vi "T_step_Kelvinox.vi"   [LabVIEW 2019]
uses:
  Global/Global Variables/global.vi
  Instrument_Setup.vi
  Global/Global Variables/Data_Display_global.vi
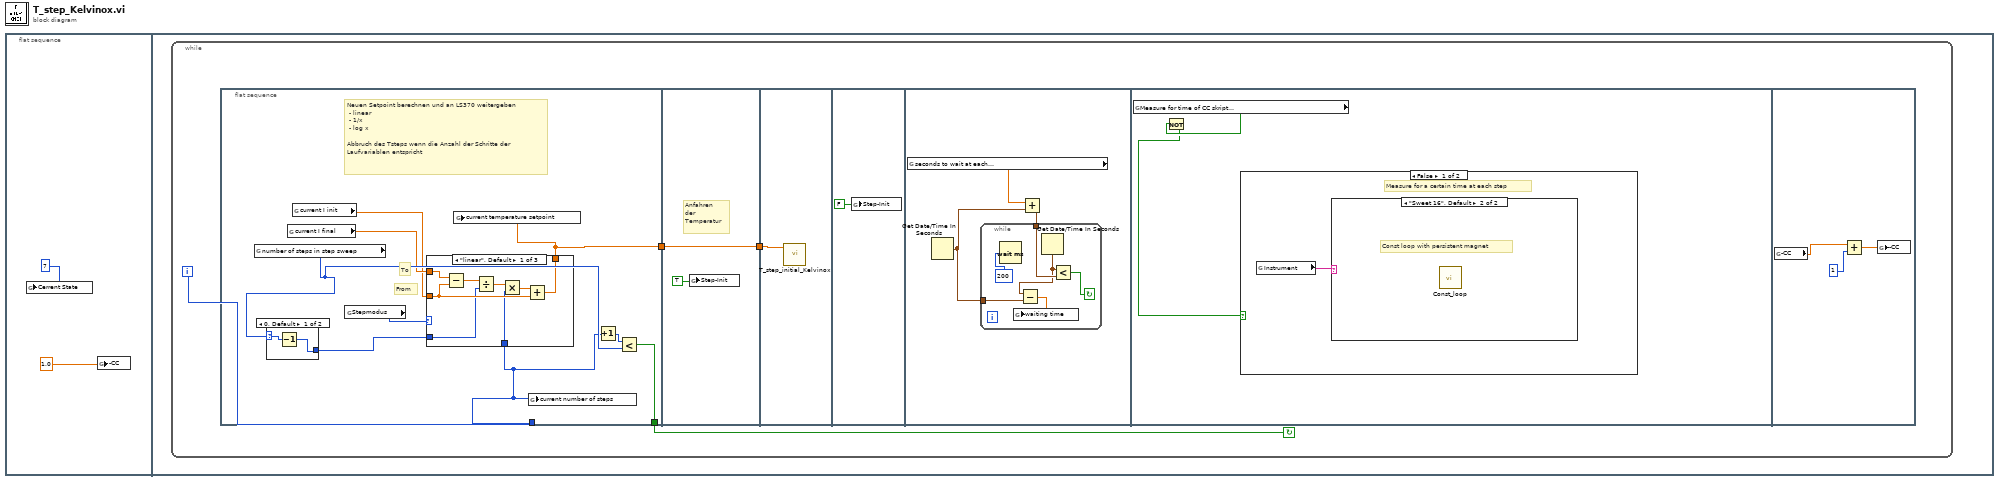
[diagram p0: block diagram]
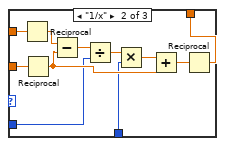
[diagram p3: hidden frame]
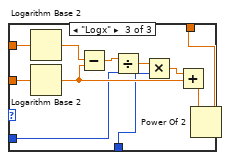
[diagram p4: hidden frame]
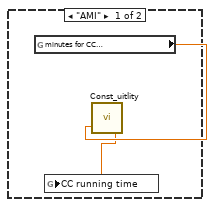
[diagram p5: hidden frame]
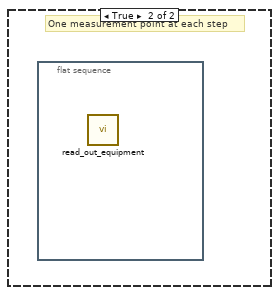
[diagram p6: hidden frame]
diagram:
  n1 = flat-sequence {
    frame #0 {
      n2 = global write "global.vi" "Cerrent State"(7) -> ()
      n3 = global write "global.vi" "-CC"(1.0) -> ()
    }
    frame #1 {
      n4 = while {
        i -> [w6]
        stop <- w5 continue-if-true
        n5 = flat-sequence {
          tunnel: w6 -> [w8]
          tunnel: [w9] -> w5
          tunnel: [w7] -> w3
          tunnel: [w49] -> w4
          tunnel: w3 -> [w49]
          tunnel: w4 -> [w51]
          frame #0 {
            # "Neuen Setpoint berechnen und an LS370 weitergeben\n - linear\n - 1/x\n - log x\n\nAbbruch des Tsteps wenn die Anzahl der Schritte der \nLaufvariablen entspricht"
            # "From"
            # "To"
            n6 = global read "global.vi" "number of steps in step sweep"() -> (w13:i32)
            n7 = case shown="0, Default" w13 {
              selector: w13 -> [w17 w18]
              tunnel: [w16 w18] -> w14
              frame 0, Default {
                n8 = Decrement(x=w17) -> (x-1=w16:i32)
              }
              frame 1 {
              }
            }
            n9 = global read "global.vi" "current I final"() -> (w11:dbl)
            n10 = global read "global.vi" "current I init"() -> (w10:dbl)
            n11 = global read "Instrument_Setup.vi" "Stepmodus"() -> (w12:enum16{"linear", "1/x", "Logx"})
            n12 = case shown="\"linear\", Default" w12 {
              tunnel: w11 -> [w26 w36 w48]
              tunnel: w10 -> [w23 w37 w47]
              tunnel: [w21 w31 w40] -> w7
              tunnel: w14 -> [w20 w28 w39]
              tunnel: w8 -> [w19 w27 w38]
              frame "linear", Default {
                n13 = Subtract(x=w26, y=w23) -> (x-y=w25:dbl)
                n14 = Divide(x=w25, y=w20) -> (x/y=w24:dbl)
                n15 = Multiply(x=w24, y=w19) -> (x*y=w22:dbl)
                n16 = Add(x=w22, y=w23) -> (x+y=w21:dbl)
              }
              frame "1/x" {
                n17 = Reciprocal(x=w36) -> (1/x=w30:dbl)
                n18 = Reciprocal(x=w37) -> (1/x=w29:dbl)
                n19 = Subtract(x=w30, y=w29) -> (x-y=w35:dbl)
                n20 = Divide(x=w35, y=w28) -> (x/y=w34:dbl)
                n21 = Multiply(x=w34, y=w27) -> (x*y=w33:dbl)
                n22 = Add(x=w33, y=w29) -> (x+y=w32:dbl)
                n23 = Reciprocal(x=w32) -> (1/x=w31:dbl)
              }
              frame "Logx" {
                n24 = Logarithm Base 2(1:w48) -> (0:w46:dbl)
                n25 = Logarithm Base 2(1:w47) -> (0:w42:dbl)
                n26 = Subtract(x=w46, y=w42) -> (x-y=w45:dbl)
                n27 = Divide(x=w45, y=w39) -> (x/y=w44:dbl)
                n28 = Multiply(x=w44, y=w38) -> (x*y=w43:dbl)
                n29 = Add(x=w43, y=w42) -> (x+y=w41:dbl)
                n30 = Power Of 2(x=w41) -> (2^x=w40:dbl)
              }
            }
            n31 = global write "Data_Display_global.vi" "current temperature setpoint"(w7) -> ()
            n32 = global write "Data_Display_global.vi" "current number of steps"(w8) -> ()
            n33 = Increment(x=w8) -> (x+1=w15:i32)
            n34 = Less?(x=w15, y=w13) -> (x < y?=w9:bool)
          }
          frame #1 {
            # "Anfahren \nder \nTemperatur"
            n35 = global write "global.vi" "Step-Init"(TRUE) -> ()
          }
          frame #2 {
            n36 = call "T_step_initial_Kelvinox.vi"("Current T Setpoint (K)"=w51) -> ()  [unwired: 3 in]
          }
          frame #3 {
            n37 = global write "global.vi" "Step-Init"(FALSE) -> ()
          }
          frame #4 {
            n38 = global read "Instrument_Setup.vi" "seconds to wait at each\nfield step in a step sweep"() -> (w53:dbl)
            n39 = Get Date/Time In Seconds() -> (seconds since 1Jan1904=w54:timestamp)
            n40 = Add(x=w53, y=w54) -> (x+y=w55:timestamp)
            n41 = while {
              tunnel: w55 -> [w61]
              tunnel: w54 -> [w57]
              stop <- w60 continue-if-true
              n42 = Wait (ms)(milliseconds to wait=u32 200) -> ()  [unwired: 1 out]
              n43 = Get Date/Time In Seconds() -> (seconds since 1Jan1904=w58:timestamp)
              n44 = Subtract(x=w58, y=w57) -> (x-y=w56:dbl)
              n45 = global write "Data_Display_global.vi" "waiting time"(w56) -> ()
              n46 = Less?(x=w58, y=w61) -> (x < y?=w60:bool)
            }
          }
          frame #5 {
            n47 = global read "Instrument_Setup.vi" "Measure for time of CC skript\nat each field step point"() -> (w63:bool)
            n48 = Not(x=w63) -> (.not. x?=w62:bool)
            n49 = case shown="False" w62 {
              frame False {
                # "Measure for a certain time at each step"
                n50 = global read "Instrument_Setup.vi" "Instrument"() -> (w64:string)
                n51 = case shown="\"Sweet 16\", Default" w64 {
                  frame "AMI" {
                    n52 = global read "Instrument_Setup.vi" "minutes for CC\nto run"() -> (w66:dbl)
                    n53 = call "Const_uitlity.vi"("Duration"=w66) -> ("Minutes passed"=w65:dbl)  [unwired: 1 in]
                    n54 = global write "Data_Display_global.vi" "CC running time"(w65) -> ()
                  }
                  frame "Sweet 16", Default {
                    # "Const loop with persistent magnet"
                    n55 = call "Const_loop.vi"() -> ()  [unwired: 4 in]
                  }
                }
              }
              frame True {
                # "One measurement point at each step"
                n56 = flat-sequence {
                  frame #0 {
                    n57 = call "read_out_equipment.vi"() -> ()  [unwired: 1 in]
                  }
                }
              }
            }
          }
          frame #6 {
            n58 = global read "global.vi" "-CC"() -> (w69:dbl)
            n59 = Add(x=w69, y=1) -> (x+y=w67:dbl)
            n60 = global write "global.vi" "-CC"(w67) -> ()
          }
        }
      }
    }
  }
